vi "LTS300CConnectMove.vi"() -> ()   [LabVIEW 2023]
uses:
  C:/Users/fmovagharnemati/OneDrive - THORLABS Inc/Desktop/github/LTS300CM/Thorlabs.MotionControl.Controls.dll
  github/LTS300CM/Thorlabs.MotionControl.Controls.dll
  C:/Users/fmovagharnemati/OneDrive - THORLABS Inc/Desktop/github/LTS300CM/Thorlabs.MotionControl.IntegratedStepperMotorsCLI.dll
  github/LTS300CM/Thorlabs.MotionControl.IntegratedStepperMotorsCLI.dll
panel:
  in  "position":dbl
  in  "Disconnect":bool
  in  "Move To Position":bool
  in  "SerialNumber":string
  in  "LongTravelStageControl":refnum<k24>(container)
  # "Thorlabs Hardware: LTS300C - 300 mm Translation Stage with Stepper Motor, Integrated Controller\nhttps://www.thorlabs.com/thorproduct.cfm?partnumber=LTS300C\n\nDescription: This VI will enable you to communicate with LTC300C integrated controller stepper motor stage. \n\nInstructions: \n1) Connect your LTC300C  device to your PC & power the device, ensuring your stage/actutator is connected. For full device setup, the device product manual can be found on our website.\n2) Enter the device serial number.\n3) Ensure the device move path is clear for homing and movement.\n4) Click 'Run' in the LabVIEW Toolbar which will attempt a connection, enable the device, and home.\n5) Await for device to be be available, and to have finished homing (Home indicator in control panel should be green).\n6) Input desired position,and press the associated button to initiate the move.\n7) To end the Program click 'STOP'."
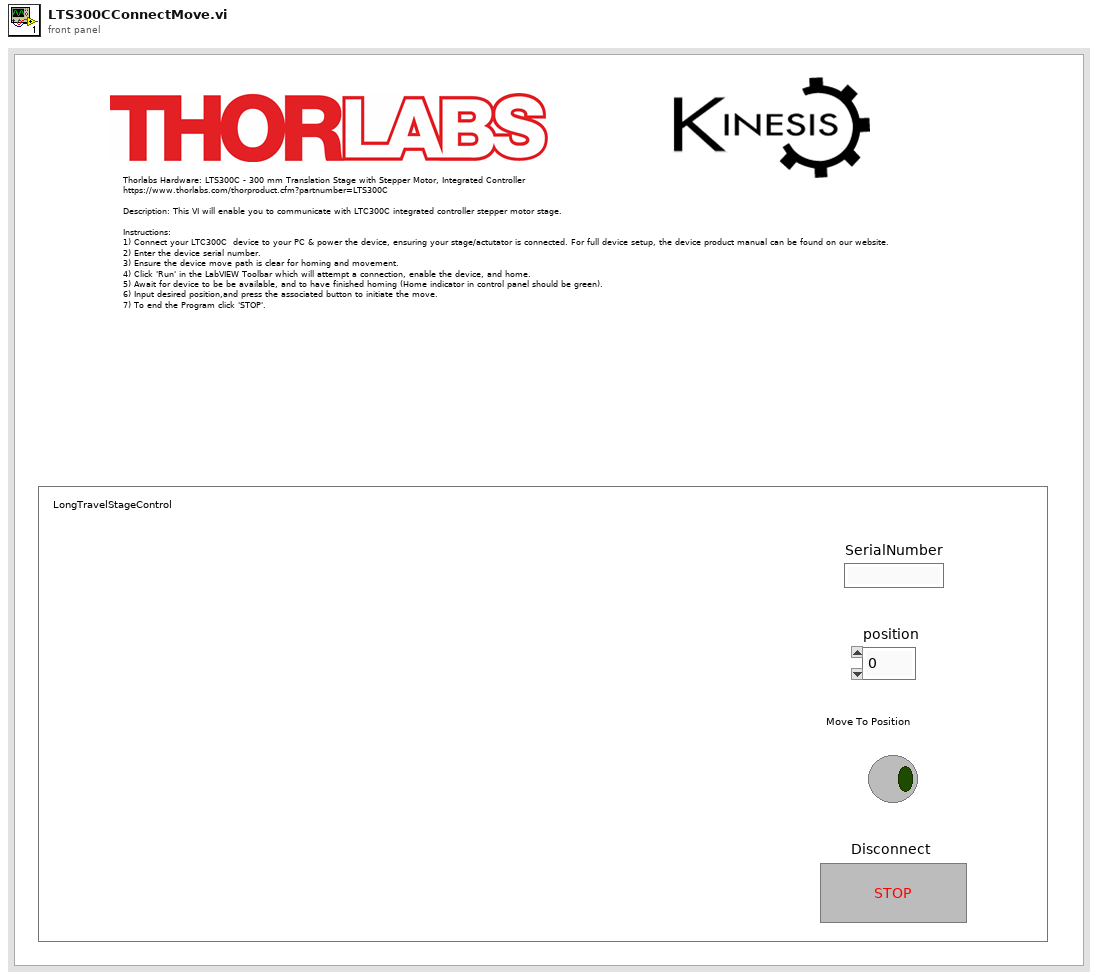
[diagram p1: front panel]
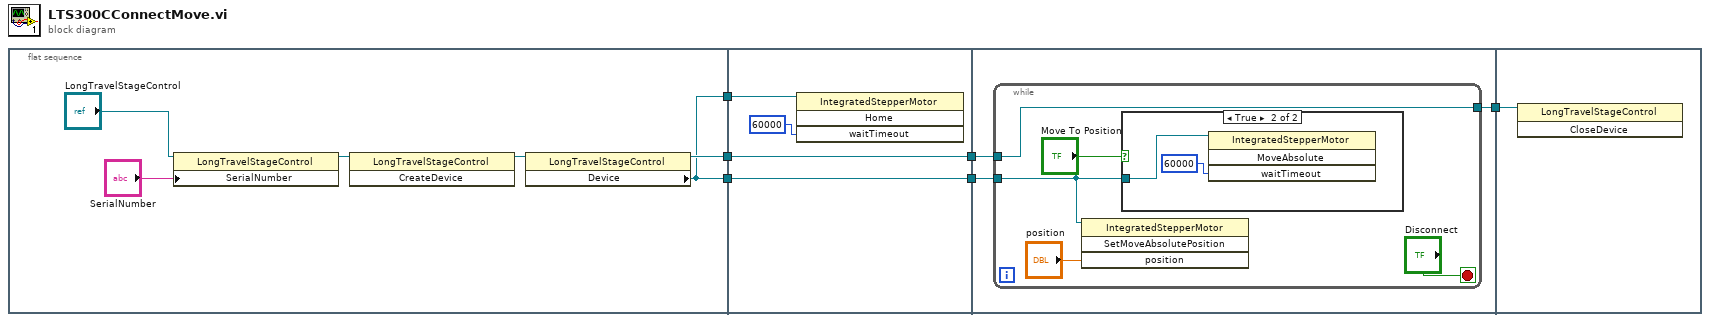
[diagram p0: block diagram]
diagram:
  n1 = flat-sequence {
    tunnel: [w8] -> w4
    tunnel: [w7] -> w3
    tunnel: [w7] -> w1
    tunnel: [w15] -> w5
    tunnel: w4 -> [w15]
    tunnel: w3 -> [w14]
    tunnel: [w13] -> w2
    tunnel: w1 -> [w13]
    tunnel: [w19] -> w6
    tunnel: w5 -> [w18]
    tunnel: w2 -> [w17]
    tunnel: w6 -> [w27]
    frame #0 {
      n2 = property class="LongTravelStageControl"(reference="LongTravelStageControl", "SerialNumber"="SerialNumber") -> (reference out=w11:refnum<k24>)  [unwired: 1 in, 1 out]
      n3 = invoke class="LongTravelStageControl" method="CreateDevice"(reference=w11) -> (reference out=w12:refnum<k24>)  [unwired: 2 in, 2 out]
      n4 = property class="LongTravelStageControl"(reference=w12) -> (reference out=w8:refnum<k24>, "Device"=w7:refnum<k24>)  [unwired: 1 in, 1 out]
    }
    frame #1 {
      n5 = invoke class="IntegratedStepperMotor" method="Home"(reference=w14, "waitTimeout"=60000) -> ()  [unwired: 2 in, 4 out]
    }
    frame #2 {
      n6 = while {
        tunnel: w18 -> [w22]
        tunnel: [w22] -> w19
        tunnel: w17 -> [w20]
        stop <- "Disconnect" stop-if-true
        n7 = invoke class="IntegratedStepperMotor" method="SetMoveAbsolutePosition"(reference=w20, "position"="position") -> ()  [unwired: 2 in, 4 out]
        n8 = case shown="True" "Move To Position" {
          tunnel: w20 -> [_ w25]
          frame False {
          }
          frame True {
            n9 = invoke class="IntegratedStepperMotor" method="MoveAbsolute"(reference=w25, "waitTimeout"=60000) -> ()  [unwired: 2 in, 4 out]
          }
        }
      }
    }
    frame #3 {
      n10 = invoke class="LongTravelStageControl" method="CloseDevice"(reference=w27) -> ()  [unwired: 2 in, 3 out]
    }
  }
